vi "Engine-RPC-SyncPumpB.vi"(8 "Error In":errorcluster, 11 "DSI Reference":refnum<class "DCM-DSI.lvclass">) -> (0 "Error Out":errorcluster, 3 "DSI Reference":refnum<class "DCM-DSI.lvclass">)   [LabVIEW 2016, in "DSI-RT.lvlib"]
uses:
  DSI-RT.lvlib
  Classes/DCM-DSI/DCM-DSI.lvclass
  Shared/Typedefs/Engine-RPC-Sync-Indicators.ctl
  <vilib>/addons/Software Calibration Management/xSCM/Controls/TBL2D.ctl
  <vilib>/Powertrain Controls/Device Drivers/DCM/Rev0/RT/DCM - RT.lvclass/DCM - RT.ctl
  <vilib>/Powertrain Controls/Device Drivers/DCM/Rev0/RT/Read Max CAD.vi
  Classes/DCM-DSI/Read DiffIO Results.vi
  Classes/DCM-DSI/Read DCM Ref.vi
  Classes/DCM-DSI/Read EPTx Data.vi
  Classes/DCM-DSI/Read Channels.vi
  Classes/DCM-DSI/Read dt.vi
  Classes/DCM-DSI/Write Pump-B Command.vi
  <vilib>/Powertrain Controls/Device Drivers/DCM/Rev0/RT/DCM - RT.lvclass
  <vilib>/addons/Software Calibration Management/xSCM/FaultPoint.xnode
  <vilib>/addons/Software Calibration Management/xSCM/CalPoint.xnode
  <vilib>/addons/Software Calibration Management/xSCM/Controls/TLU2D.ctl
  <vilib>/addons/Software Calibration Management/xSCM/ni_scm.dll
  <vilib>/addons/Software Calibration Management/xSCM/SCM-API.lvlib
  Shared/DSI-Shared.lvlib
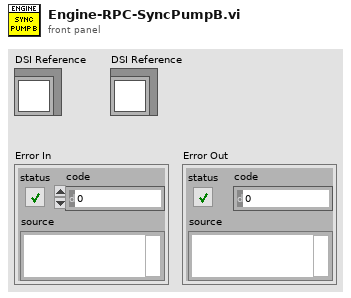
[diagram p1: front panel]
types:
  T1 = typedef "DSI-Shared.lvlib/Engine-RPC-Sync-Indicators.ctl" = cluster{"Duration":cluster{"Duration_Output":sgl, "PID_Output":sgl}, "EPT Mode":cluster{"Sync-A_Timing":sgl, "Sync-A_CamAdv":sgl}, "TMP Mode":cluster{"Sync-A_Delay":sgl, "Sync-A_Period":sgl}}
  T2 = cluster{"PID_Kp":sgl, "PID_Ti":sgl, "PID_Td":sgl, "PID_FF":sgl, "Non-PID_FF":sgl, "PID_Min":sgl, "PID_Max":sgl}
  T3 = typedef "DCM - RT - Diff IO.lvlib/Results.ctl" = cluster{"Capture [DBTDC]":sgl, "Capture Error":bool, "Frequency [Hz]":sgl, "Duty Cycle [%]":sgl, "PWM Stopped":bool}
  T4 = typedef "EPTx - RevA - RT.lvlib/EPTxData.ctl" = cluster{"Sync":bool, "CurrentCAD":sgl, "Speed [RPM]":sgl, "Config":bool, "Rcvg Primary":bool, "Stall":bool, "Overflow":bool, "Ratio Error":bool, "Pattern Error":bool, "Aux Warning":bool, "Watchdog Error":bool}
  T5 = typedef "DCM-DSI.lvclass/Channel.ctl" = cluster{"Name":string, "Unit":string, "Value":sgl}
  T6 = typedef "DSI-Shared.lvlib/Engine-Channel.ctl" = cluster{"Name":string, "Unit":string, "Value":sgl}
  T7 = typedef "SCM-API.lvlib/TBL2D.ctl" = cluster{"X":sgl[], "Y":sgl[], "Z":sgl[][]}
  T8 = typedef "SCM-API.lvlib/TLU2D.ctl" = cluster{"X":sgl, "Y":sgl, "Z":sgl}
  T9 = cluster{"Duration":cluster{"Dur_Max":sgl, "Dur_Min":sgl, "Dur_ManE":bool, "Dur_Man":sgl}, "Timing":cluster{"WindowStart":sgl, "WindowEnd":sgl, "EndAngle?":bool, "DurAngle_Max":sgl, "MinOffTime":sgl}}
  T10 = cluster{"Dur_Max":sgl, "Dur_Min":sgl, "Dur_ManE":bool, "Dur_Man":sgl}
  T11 = cluster{"WindowStart":sgl, "WindowEnd":sgl, "EndAngle?":bool, "DurAngle_Max":sgl, "MinOffTime":sgl}
  T12 = cluster{"ProportionalAction":sgl, "IntegralAction":sgl, "DerivativeAction":sgl}
  T13 = enum8{"Unused", "User OS", "Diff IO 1", "Diff IO 2", "Diff IO 3", "Diff IO 4", "Diff IO 5", "Diff IO 6", "Diff IO 7", "Diff IO 8", "Aux 1", "Aux 2", "Aux 3", "Aux 4", "Aux 5", "Aux 6", "Aux 7", "Aux 8", "Aux 9", "Aux 10", "Aux 11", "Aux 12", "Aux 13", "Aux 14", "Aux 15", "Aux 16"}
  T14 = cluster{"Value":enum8{"Unused", "User OS", "Diff IO 1", "Diff IO 2", "Diff IO 3", "Diff IO 4", "Diff IO 5", "Diff IO 6", "Diff IO 7", "Diff IO 8", "Aux 1", "Aux 2", "Aux 3", "Aux 4", "Aux 5", "Aux 6", "Aux 7", "Aux 8", "Aux 9", "Aux 10", "Aux 11", "Aux 12", "Aux 13", "Aux 14", "Aux 15", "Aux 16"}, "Value":sgl}
  T15 = cluster{"Value":sgl, "Value":sgl, "Duration_Output":sgl}
  T16 = typedef "DCM - RT - DI.lvlib/Command.ctl" = cluster{"Mode":T17, "Digital Input":T18, "Default Profile Index":u8, "Cal Freq [Hz]":sgl, "Cal Duration [s]":sgl, "Cal Increment [s]":sgl, "Cal Pulses":u16, "TMP Command Sequence":T19[], "EPT TDC Offset [CAD]":sgl, "EPT Window Start [DBTDC]":sgl, "EPT Window End [DBTDC]":sgl, "EPT Angles":T20[], "EPT Skip Fire":bool, "EPT Skip Index":u8, "EPT Precharge Duration [s]":sgl, "EPT Precharge Profile Index":u8}
  T17 = typedef "DCM - FPGA - DI.lvlib/Mode.ctl" = enum8{"Off", "Direct", "Calibration", "Triggered Multi-Pulse", "Engine Position Tracking"}
  T18 = typedef "DCM - FPGA.lvlib/Digital Channel.ctl" = enum8{"Unused", "User OS", "Diff IO 1", "Diff IO 2", "Diff IO 3", "Diff IO 4", "Diff IO 5", "Diff IO 6", "Diff IO 7", "Diff IO 8", "Aux 1", "Aux 2", "Aux 3", "Aux 4", "Aux 5", "Aux 6", "Aux 7", "Aux 8", "Aux 9", "Aux 10", "Aux 11", "Aux 12", "Aux 13", "Aux 14", "Aux 15", "Aux 16"}
  T19 = typedef "DCM - RT - DI.lvlib/Command Sequence.ctl" = cluster{"Duration [s]":sgl, "Level":bool, "Run/Stop":bool, "Profile Index":u8}
  T20 = typedef "DCM - RT - DI.lvlib/Angle Control.ctl" = cluster{"Enable":bool, "Timing [DBTDC]":sgl, "Duration [s]":sgl, "Profile Index":u8}
  T21 = cluster{"Sync-A_Timing":sgl, "Sync-A_CamAdv":sgl}
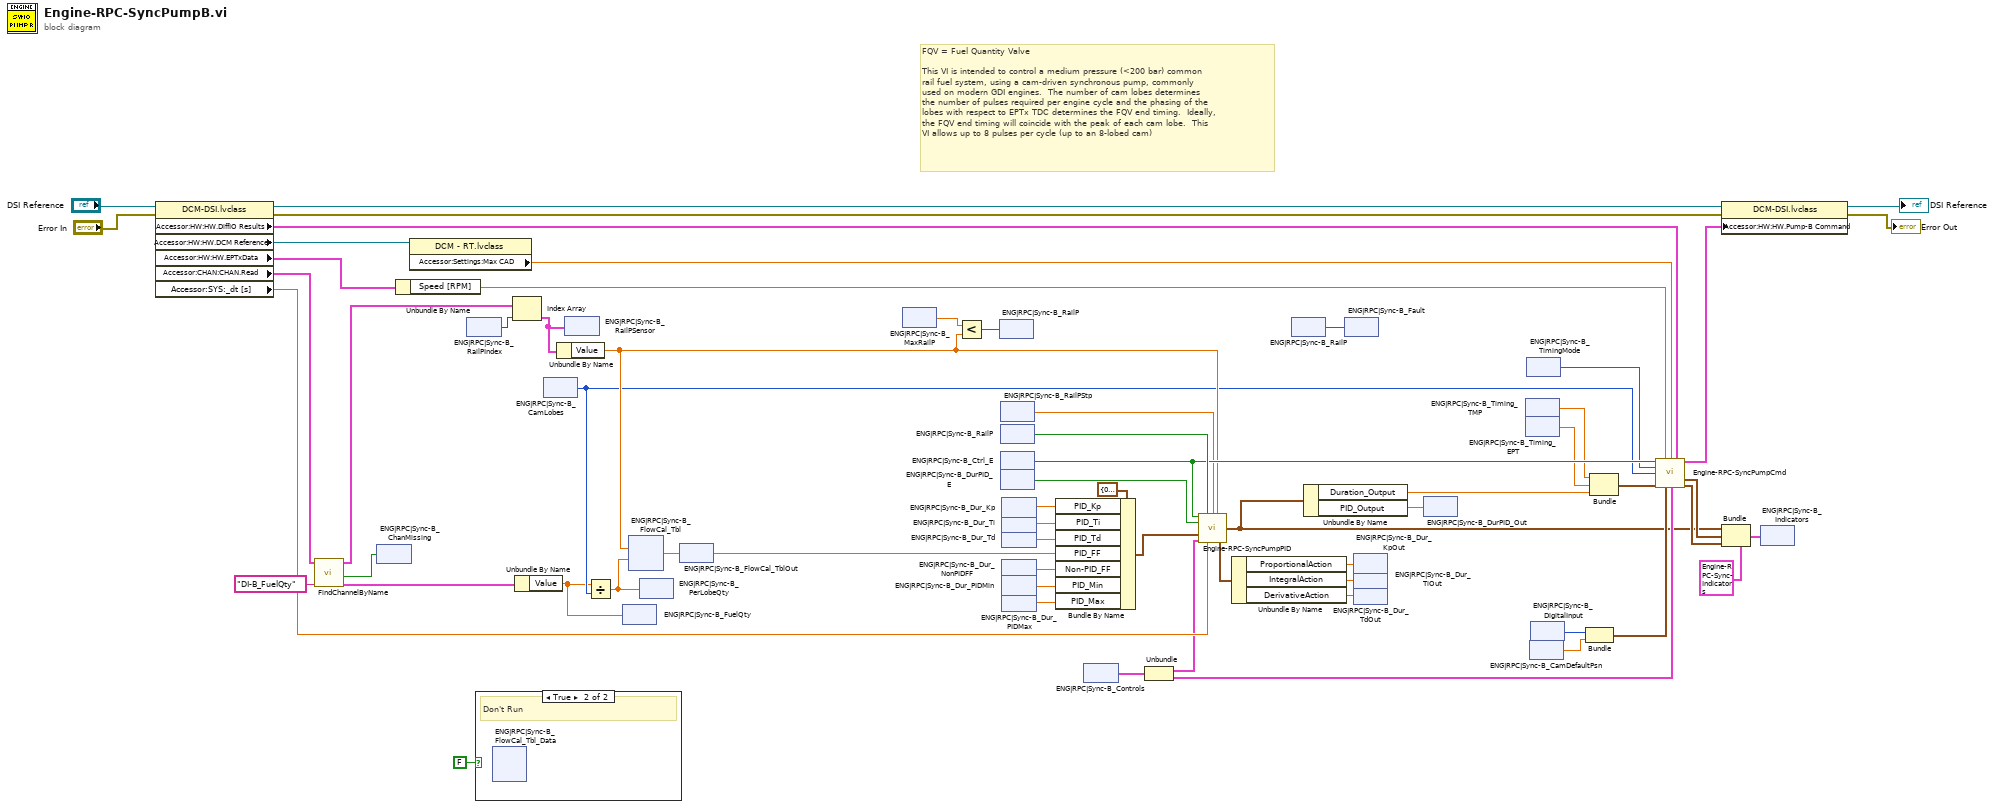
[diagram p0: block diagram]
diagram:
  # "FQV = Fuel Quantity Valve\n\nThis VI is intended to control a medium pressure (<200 bar) common\nrail fuel system, using a cam-driven synchronous pump, commonly\nused on modern GDI engines.  The number of cam lobes determines \nthe number of pulses required per engine cycle and the phasing of the\nlobes with respect to EPTx TDC determines the FQV end timing.  Ideally,\nthe FQV end timing will coincide with the peak of each cam lobe.  This\nVI allows up to 8 pulses per cycle (up to an 8-lobed cam)"
  n1 = property class="DCM-DSI.lvclass"(reference="DSI Reference", error in="Error In") -> (reference out=w45:refnum<class "DCM-DSI.lvclass">, error out=w44:errorcluster, "Accessor:HW:HW.DiffIO Results"=w31:T3[], "Accessor:HW:HW.DCM Reference"=w32:refnum<class "DCM - RT.lvclass">, "Accessor:HW:HW.EPTxData"=w43:T4, "Accessor:CHAN:CHAN.Read"=w8:T5[], "Accessor:SYS:_dt [s]"=w40:sgl)
  n2 = call "FindChannelByName.vi"("Name"="DI-B_FuelQty", "CTRL.Channels in"=w8) -> ("Channel"=w9:T6, "Searching"=w6:bool, "CTRL.Channels out"=w4:T6[])  [unwired: 6 in, 1 out]
  n3 = xnode "ENG|RPC|Sync-B_ChanMissing"("Fault"=w6) -> ()
  n4 = Unbundle By Name(w43) -> ("Speed [RPM]"=w36:sgl)
  n5 = property class="DCM - RT.lvclass"(reference=w32) -> ("Accessor:Settings:Max CAD"=w33:sgl)  [unwired: 1 in, 2 out]
  n6 = xnode "ENG|RPC|Sync-B_RailPIndex"() -> ("Value"=w2:i32)
  n7 = case shown="True" FALSE {
    frame False {
    }
    frame True {
      # "Don't Run"
      n8 = xnode "ENG|RPC|Sync-B_FlowCal_Tbl_Data"() -> ()  [unwired: 1 out]
    }
  }
  n9 = Index Array(array=w4, index=w2) -> (element=w3:T6)
  n10 = Unbundle By Name(w9) -> ("Value"=w11:sgl)
  n11 = xnode "ENG|RPC|Sync-B_CamLobes"() -> ("Value"=w21:u8)
  n12 = Unbundle By Name(w3) -> ("Value"=w22:sgl)
  n13 = xnode "ENG|RPC|Sync-B_RailPSensor"("Value"=w3) -> ()
  n14 = Divide(x=w11, y=w21) -> (x/y=w38:sgl)
  n15 = xnode "ENG|RPC|Sync-B_FuelQty"("Value"=w11) -> ()
  n16 = xnode "ENG|RPC|Sync-B_FlowCal_Tbl"("Y Index"=w38, "X Index"=w22) -> ("Z"=w46:sgl)
  n17 = xnode "ENG|RPC|Sync-B_PerLobeQty"("Value"=w38) -> ()
  n18 = xnode "ENG|RPC|Sync-B_FlowCal_TblOut"("Value"=w46) -> ()
  n19 = xnode "ENG|RPC|Sync-B_MaxRailP"() -> ("Value"=w23:sgl)
  n20 = Less?(x=w23, y=w22) -> (x < y?=w42:bool)
  n21 = xnode "ENG|RPC|Sync-B_RailP"("Fault"=w42) -> ()
  n22 = xnode "ENG|RPC|Sync-B_RailPStp"() -> ("Value"=w13:sgl)
  n23 = xnode "ENG|RPC|Sync-B_RailP"() -> ("Fault"=w41:bool)
  n24 = xnode "ENG|RPC|Sync-B_Ctrl_E"() -> ("Value"=w37:bool)
  n25 = xnode "ENG|RPC|Sync-B_DurPID_E"() -> ("Value"=w47:bool)
  n26 = xnode "ENG|RPC|Sync-B_Dur_Kp"() -> ("Value"=w51:sgl)
  n27 = xnode "ENG|RPC|Sync-B_Dur_Ti"() -> ("Value"=w52:sgl)
  n28 = xnode "ENG|RPC|Sync-B_Dur_Td"() -> ("Value"=w53:sgl)
  n29 = xnode "ENG|RPC|Sync-B_Dur_NonPIDFF"() -> ("Value"=w39:sgl)
  n30 = xnode "ENG|RPC|Sync-B_Dur_PIDMin"() -> ("Value"=w54:sgl)
  n31 = xnode "ENG|RPC|Sync-B_Dur_PIDMax"() -> ("Value"=w55:sgl)
  n32 = Bundle By Name(cluster=T2 {"PID_Kp"=0.0, "PID_Ti"=0.01, "PID_Td"=0.0, "PID_FF"=0.0, "Non-PID_FF"=0.0, "PID_Min"=-100.0, "PID_Max"=100.0} ("PID Settings"), "PID_Kp"=w51, "PID_Ti"=w52, "PID_Td"=w53, "PID_FF"=w46, "Non-PID_FF"=w39, "PID_Min"=w54, "PID_Max"=w55) -> (w48:T2)
  n33 = xnode "ENG|RPC|Sync-B_Controls"() -> ("Value"=w20:T9)
  n34 = Unbundle(w20) -> ("Duration"=w19:T10, "Timing"=w18:T11)
  n35 = call "Engine-RPC-SyncPumpPID.vi"("Control Enable"=w37, "Fault Input"=w41, "Rail Press Setpoint"=w13, "Rail Pressure"=w22, "PID Enable"=w47, "PID Settings"=w48, "Output Management Controls"=w19, "dt (s)"=w40) -> ("Output"=w15:cluster{"Duration_Output":sgl, "PID_Output":sgl}, "PID_Action_Output"=w50:T12)  [unwired: 6 in]
  n36 = Unbundle By Name(w50) -> ("ProportionalAction"=w58:sgl, "IntegralAction"=w57:sgl, "DerivativeAction"=w56:sgl)
  n37 = xnode "ENG|RPC|Sync-B_RailP"() -> ("Fault"=w7:bool)
  n38 = Unbundle By Name(w15) -> ("Duration_Output"=w25:sgl, "PID_Output"=w12:sgl)
  n39 = xnode "ENG|RPC|Sync-B_Fault"("Value"=w7) -> ()
  n40 = xnode "ENG|RPC|Sync-B_Dur_KpOut"("Value"=w58) -> ()
  n41 = xnode "ENG|RPC|Sync-B_Dur_TiOut"("Value"=w57) -> ()
  n42 = xnode "ENG|RPC|Sync-B_Dur_TdOut"("Value"=w56) -> ()
  n43 = xnode "ENG|RPC|Sync-B_DurPID_Out"("Value"=w12) -> ()
  n44 = xnode "ENG|RPC|Sync-B_Timing_TMP"() -> ("Value"=w27:sgl)
  n45 = xnode "ENG|RPC|Sync-B_Timing_EPT"() -> ("Value"=w26:sgl)
  n46 = xnode "ENG|RPC|Sync-B_TimingMode"() -> ("Value"=w28:bool)
  n47 = xnode "ENG|RPC|Sync-B_CamDefaultPsn"() -> ("Value"=w34:sgl)
  n48 = xnode "ENG|RPC|Sync-B_DigitalInput"() -> ("Value"=w35:T13)
  n49 = Bundle("Value"=w35, "Value"=w34) -> (w29:T14)  [unwired: 1 in]
  n50 = Bundle("Value"=w27, "Value"=w26, "Duration_Output"=w25) -> (w24:T15)  [unwired: 1 in]
  n51 = call "Engine-RPC-SyncPumpCmd.vi"("FQV Enable"=w37, "Engine Speed [RPM]"=w36, "MaxCAD"=w33, "HW.DiffIO Results"=w31, "Mode [T=Trig,F=EPT]"=w28, "Cam Lobes"=w21, "Command"=w24, "DigitalInputSettings"=w29, "EPT Mode Settings"=w18) -> ("Pump Command"=w30:T16, "EPT Mode Output"=w17:T21, "TMP Mode Output"=w16:cluster{"Sync-A_Delay":sgl, "Sync-A_Period":sgl})  [unwired: 4 in]
  n52 = property class="DCM-DSI.lvclass"(reference=w45, error in=w44, "Accessor:HW:HW.Pump-B Command"=w30) -> (reference out=→"DSI Reference":refnum<class "DCM-DSI.lvclass">, error out=→"Error Out":errorcluster)
  n53 = Bundle(cluster=T1 {"Duration"={"Duration_Output"=0.0, "PID_Output"=0.0}, "EPT Mode"={"Sync-A_Timing"=0.0, "Sync-A_CamAdv"=0.0}, "TMP Mode"={"Sync-A_Delay"=0.0, "Sync-A_Period"=0.0}} ("Sync-A_Results"), "Duration"=w15, "EPT Mode"=w17, "TMP Mode"=w16) -> (w14:T1)
  n54 = xnode "ENG|RPC|Sync-B_Indicators"("Value"=w14) -> ()
